vi "automatic_abort.vi"(7 "references":T1, 8 "error in (no error)":errorcluster) -> (0 "error out":errorcluster)   [LabVIEW 2015, in "lv-recipe-machine.lvlib"]
uses:
  lv-recipe-machine.lvlib
  _controls/references.ctl
  _controls/input.ctl
  _controls/input_command.ctl
  _controls/output.ctl
  _controls/data.ctl
  _controls/configuration.ctl
  _controls/recipe_data.ctl
  _controls/mode.ctl
  _controls/manual_state.ctl
  _controls/automatic_state.ctl
  _controls/recipe_step.ctl
  <userlib>/antonio-alexander/lv-waitgroup/public/_controls/api_waitgroup.ctl
  _controls/change.ctl
  _controls/status.ctl
  _controls/error.ctl
  <userlib>/antonio-alexander/lv-waitgroup/lv-waitgroup.lvlib
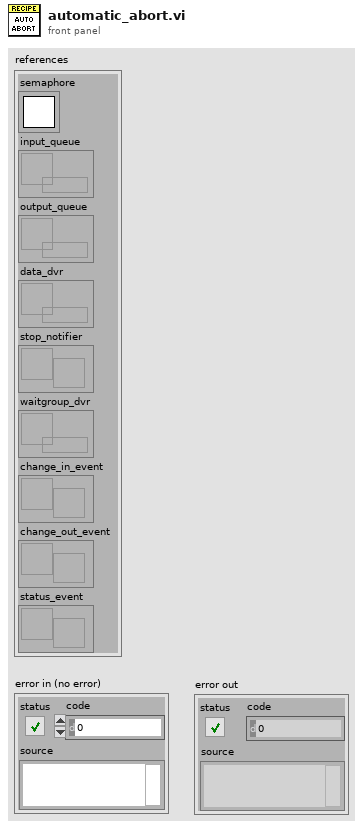
[diagram p1: front panel]
types:
  T1 = typedef "lv-recipe-machine.lvlib/references.ctl" = cluster{"semaphore":T2, "input_queue":refnum<queue>, "output_queue":refnum<queue>, "data_dvr":refnum<data-value>, "stop_notifier":refnum<notifier>, "waitgroup_dvr":refnum<data-value>, "change_in_event":refnum<user-event>, "change_out_event":refnum<user-event>, "status_event":refnum<user-event>}
  T2 = typedef "Semaphore RefNum" = refnum<k1>
  T3 = typedef "lv-recipe-machine.lvlib/error.ctl" = enum16{"<error>", "bad_command", "command_queue_timeout", "stop_notifier_timeout", "die_command_timeout", "not_in_manual_mode", "not_in_automatic_mode", "not_in_automatic_idle", "not_in_automatic_running", "not_in_automatic_paused", "automatic_step_not_found", "manual_step_not_found", "<null>"}
  T4 = typedef "lv-recipe-machine.lvlib/automatic_state.ctl" = enum16{"<automatic_state>", "failed", "idle", "running", "paused", "transition", "stopped", "<null>"}
  T5 = typedef "lv-recipe-machine.lvlib/data.ctl" = cluster{"configuration":T6, "working":cluster{"recipe_data":T7, "api_waitgroup":T11}}
  T6 = typedef "lv-recipe-machine.lvlib/configuration.ctl" = cluster{"max_processes":i32}
  T7 = typedef "lv-recipe-machine.lvlib/recipe_data.ctl" = cluster{"mode":T8, "manual_state":T9, "automatic_state":T4, "previous_automatic_state":T4, "error":errorcluster, "manual":cluster{"step_action":string, "data":variant, "actions":variant}, "automatic":cluster{"data":variant, "steps":variant, "criteria":variant, "transition":string, "index":i32, "recipe []":T10[]}}
  T8 = typedef "lv-recipe-machine.lvlib/mode.ctl" = enum16{"<mode>", "manual", "automatic", "<null>"}
  T9 = typedef "lv-recipe-machine.lvlib/manual_state.ctl" = enum16{"<manual_state>", "failed", "action", "running", "idle", "<null>"}
  T10 = typedef "lv-recipe-machine.lvlib/recipe_step.ctl" = cluster{"step":string, "data":variant}
  T11 = typedef "lv-waitgroup.lvlib/api_waitgroup.ctl" = cluster{"waitgroups":refnum<data-value>, "waitgroup":string}
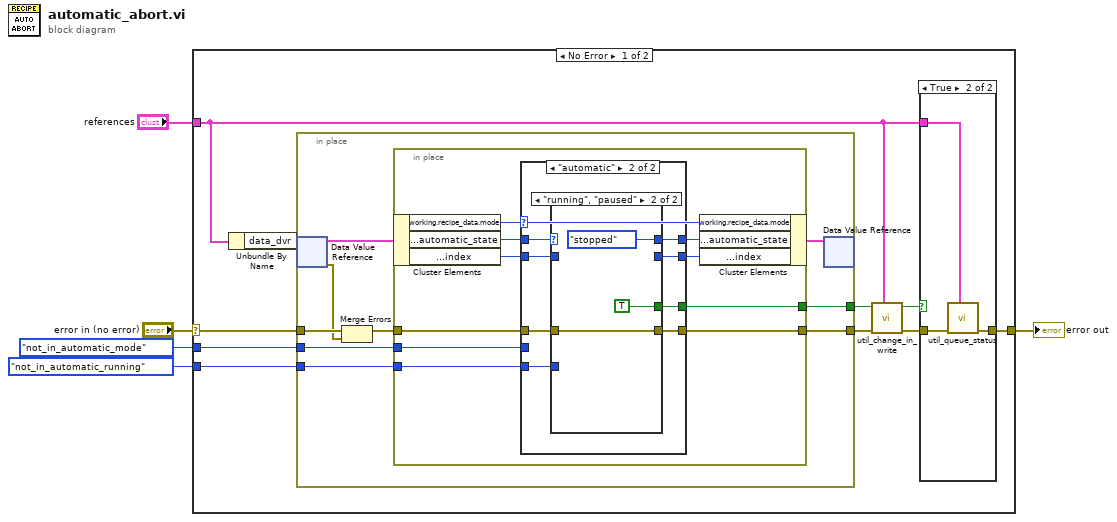
[diagram p0: block diagram]
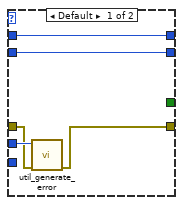
[diagram p2: hidden frame]
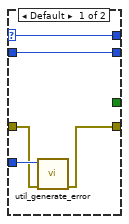
[diagram p3: hidden frame]
diagram:
  n1 = case shown="No Error" "error in (no error)" {
    selector: "error in (no error)" -> [w13 w59]
    tunnel: [w8 w59] -> w4
    tunnel: "references" -> [w7 _]
    tunnel: error."not_in_automatic_mode" ("error") -> [w12 _]
    tunnel: error."not_in_automatic_running" ("error") -> [w11 _]
    frame No Error {
      n2 = Unbundle By Name(w7) -> ("data_dvr"=w14:refnum<data-value>)
      n3 = in-place {
        in-place-border: w13 -> [w23]
        in-place-border: w12 -> [w18]
        in-place-border: [w17] -> w9
        in-place-border: w11 -> [w16]
        in-place-border: [w15] -> w6
        n4 = in-place-dvr #1(w14) -> (w21:T5, w22:errorcluster)
        n5 = Merge Errors(w23, w22) -> (w20:errorcluster)
        n6 = in-place {
          in-place-border: w20 -> [w31]
          in-place-border: w18 -> [w30]
          in-place-border: [w29] -> w17
          in-place-border: w16 -> [w25]
          in-place-border: [w24] -> w15
          n7 = in-place-cluster #2(w21) -> ("working.recipe_data.mode"=w28:T8, "working.recipe_data.automatic_state"=w33:T4, "working.recipe_data.automatic.index"=w32:i32)
          n8 = case shown="\"automatic\"" w28 {
            tunnel: w33 -> [w35 w45]
            tunnel: w32 -> [w34 w44]
            tunnel: w31 -> [w37 w43]
            tunnel: w30 -> [w38 _]
            tunnel: [w36 w42] -> w29
            tunnel: [w35 w40] -> w27
            tunnel: [w34 w41] -> w26
            tunnel: w25 -> [_ w46]
            tunnel: [_ w39] -> w24
            frame Default {
              n9 = call "util_generate_error.vi"("error in (no error)"=w37, "error"=w38) -> ("error out"=w36:errorcluster)  [unwired: 9 in]
            }
            frame "automatic" {
              n10 = case shown="\"running\", \"paused\"" w45 {
                selector: w45 -> [w47 _]
                tunnel: w46 -> [w51 _]
                tunnel: w44 -> [w48 _]
                tunnel: w43 -> [w50 w54]
                tunnel: [w49 w54] -> w42
                tunnel: [w48 _] -> w41
                tunnel: [w47 automatic_state."stopped" ("automatic_state")] -> w40
                tunnel: [_ TRUE] -> w39
                frame Default {
                  n11 = call "util_generate_error.vi"("error in (no error)"=w50, "error"=w51) -> ("error out"=w49:errorcluster)  [unwired: 9 in]
                }
                frame "running", "paused" {
                }
              }
            }
          }
          n12 = in-place-cluster #2("working.recipe_data.mode"=w28, "working.recipe_data.automatic_state"=w27, "working.recipe_data.automatic.index"=w26) -> (w19:T5)
        }
        n13 = in-place-dvr #1(w19) -> ()  [unwired: 2 out]
      }
      n14 = call "util_change_in_write.vi"("references"=w7, "error in (no error)"=w9, "data"=w6) -> ("error out"=w10:errorcluster)  [unwired: 8 in]
      n15 = case shown="True" w6 {
        tunnel: w10 -> [w55 w58]
        tunnel: [w55 w56] -> w8
        tunnel: w7 -> [_ w57]
        frame False {
        }
        frame True {
          n16 = call "util_queue_status.vi"("references"=w57, "error in (no error)"=w58) -> ("error out"=w56:errorcluster)  [unwired: 9 in]
        }
      }
    }
    frame Error {
    }
  }
  "error out" <- w4
